vi "shortCircuits to MB01.vi"(11 "shorted circuits":bool[](array[boolean])) -> (3 "control MB01":bool[](array[boolean]))   [LabVIEW 2018, in "MB Relay.lvlib"]
uses:
  Instrument Drivers/LV_driver_MBrelay/MB Relay.lvlib
panel:
  out "error out":errorcluster
  in  "error in (no error)":errorcluster
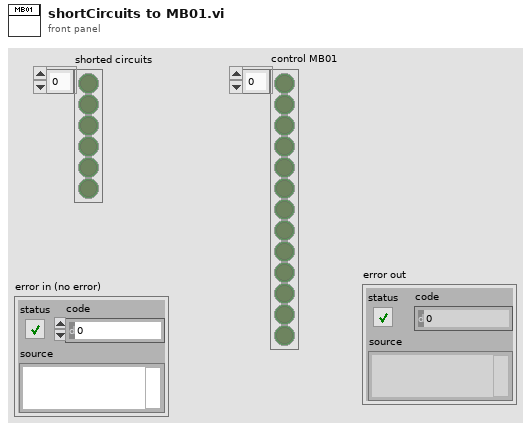
[diagram p1: front panel]
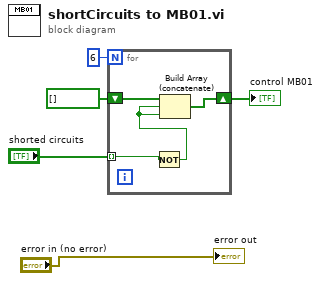
[diagram p0: block diagram]
diagram:
  n1 = for {
    N: 6 -> [_]
    tunnel: "shorted circuits" -> [w6] mode=indexing
    shift-right: [w9] -> w2
    shift-left: bool[] [] -> [w8]
    n2 = Not(x=w6) -> (.not. x?=w7:bool)
    n3 = Build Array (concatenate)(w8, w7, w7) -> (w9:bool[])
  }
  "control MB01" <- w2
  "error out" <- "error in (no error)"
